vi "Set VI Reference.vi"(8 "error in (no error)":errorcluster, 10 "VI Refnum":refnum<vi>, 11 "VI Reference Control in":refnum<class "VI Reference Control.lvclass">) -> (0 "error out":errorcluster, 3 "VI Reference Control out":refnum<class "VI Reference Control.lvclass">)   [LabVIEW 2016, in "VI Reference Control.lvclass"]
uses:
  VI Reference Control.lvclass
  C:/Users/tblair/Documents/Git Projects/Drag and Drop VI Tool/Reference Control/Reference Control.lvclass
  VI Reference Control.lvclass/VI Reference Control.ctl
  Reference Control/Reference Control.lvclass
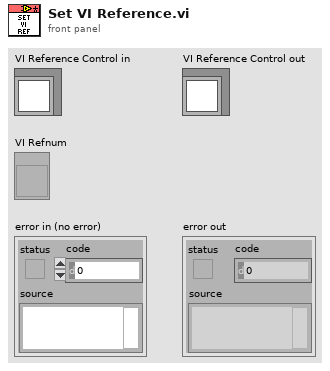
[diagram p1: front panel]
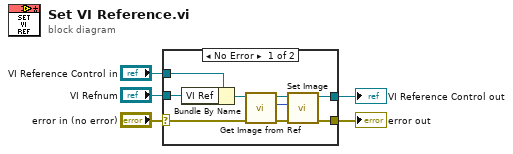
[diagram p0: block diagram]
diagram:
  n1 = case shown="No Error" "error in (no error)" {
    selector: "error in (no error)" -> [w7 w16]
    tunnel: [w6 w16] -> w4
    tunnel: [w9 w15] -> w2
    tunnel: "VI Reference Control in" -> [w14 w15]
    tunnel: "VI Refnum" -> [w13 _]
    frame No Error {
      n2 = Bundle By Name(cluster=w14, "VI Ref"=w13) -> (w12:refnum<class "VI Reference Control.lvclass">)
      n3 = call-dynamic "Get Image from Ref.vi"("error in (no error)"=w7, "VI Reference Control in"=w12) -> ("error out"=w8:errorcluster, "new picture"=w11:picture, "VI Reference Control out"=w10:refnum<class "VI Reference Control.lvclass">)  [unwired: 7 in]
      n4 = call "Set Image.vi"("error in (no error)"=w8, "Picture"=w11, "Reference Control in"=w10) -> ("error out"=w6:errorcluster, "Reference Control out"=w9:refnum<class "VI Reference Control.lvclass">)  [unwired: 7 in]
    }
    frame Error {
    }
  }
  "error out" <- w4
  "VI Reference Control out" <- w2
